vi "ReadSetLabelPosition__slk_mt.vi"(8 "error in (no error)":errorcluster, 11 "refnum in":T1) -> (0 "error out":errorcluster, 2 "set label position configure":T2={"Control Label Position"="Left Middle", "Indicator Label Position"="Right Middle", "Apply to All"=FALSE}, 3 "refnum out":T1)   [LabVIEW 2012, in "Lazyboots Menu Tool.lvlib"]
doc: "Gets configure datum of Set Label Position.\n\n<b>[Set Label Position]</b>\nControl Label Position = \"Left Middle\"\nIndicator Label Position = \"Right Middle\"\nApply to All = \"FALSE\""
uses:
  Library/Lazyboots Menu Tool.lvlib
  <vilib>/Utility/config.llb/NI_LVConfig.lvlib
  <vilib>/Utility/config.llb/Read Key (String).vi
  TypeDef/TypeDef_SetLabelPositionConfigure__slk_mt.ctl
  <vilib>/Utility/config.llb/Read Key (Boolean).vi
  <vilib>/Utility/config.llb/Config Data RefNum.ctl
panel:
  # "ReadSetLabelPosition__slk_mt.vi\nGets configure datum of Set Label Position.\n\nNOTICE -- YOU MUST LEAVE THIS NOTICE IN PLACE.\n\nCopyright (c) 2011, LIANG LIU Shawn.Liu.cn@gmail.com\nAll rights reserved.\n\nRedistribution and use in source and binary forms, with or without modification, are permitted provided that the following conditions are met:\n-Redistributions of source code must retain the above copyright notice, this list of conditions and the following disclaimer.\n-Redistributions in binary form must reproduce the above copyright notice, this list of conditions and the following disclaimer in the documentation and/or other materials provided with the distribution.\n-Neither the name of the eLp nor the names of its contributors may be used to endorse or promote products derived from this software without specific prior written permission.\n\nTHIS SOFTWARE IS PROVIDED BY THE COPYRIGHT HOLDERS AND CONTRIBUTORS \"AS IS\" AND ANY EXPRESS OR IMPLIED WARRANTIES, INCLUDING, BUT NOT LIMITED TO, THE IMPLIED WARRANTIES OF MERCHANTABILITY AND FITNESS FOR A PARTICULAR PURPOSE ARE DISCLAIMED. IN NO EVENT SHALL THE COPYRIGHT HOLDER OR CONTRIBUTORS BE LIABLE FOR ANY DIRECT, INDIRECT, INCIDENTAL, SPECIAL, EXEMPLARY, OR CONSEQUENTIAL DAMAGES (INCLUDING, BUT NOT LIMITED TO, PROCUREMENT OF SUBSTITUTE GOODS OR SERVICES; LOSS OF USE, DATA, OR PROFITS; OR BUSINESS INTERRUPTION) HOWEVER CAUSED AND ON ANY THEORY OF LIABILITY, WHETHER IN CONTRACT, STRICT LIABILITY, OR TORT (INCLUDING NEGLIGENCE OR OTHERWISE) ARISING IN ANY WAY OUT OF THE USE OF THIS SOFTWARE, EVEN IF ADVISED OF THE POSSIBILITY OF SUCH DAMAGE."
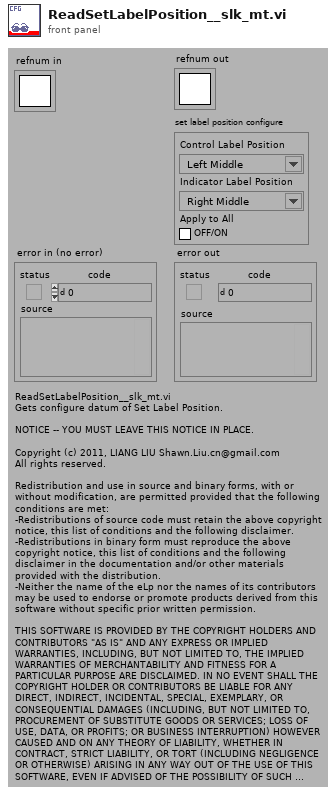
[diagram p1: front panel]
types:
  T1 = typedef "NI_LVConfig.lvlib/Config Data RefNum.ctl" = refnum<k1>
  T2 = typedef "Lazyboots Menu Tool.lvlib/TypeDef_SetLabelPositionConfigure__slk_mt.ctl" = cluster{"Control Label Position":string, "Indicator Label Position":string, "Apply to All":bool}
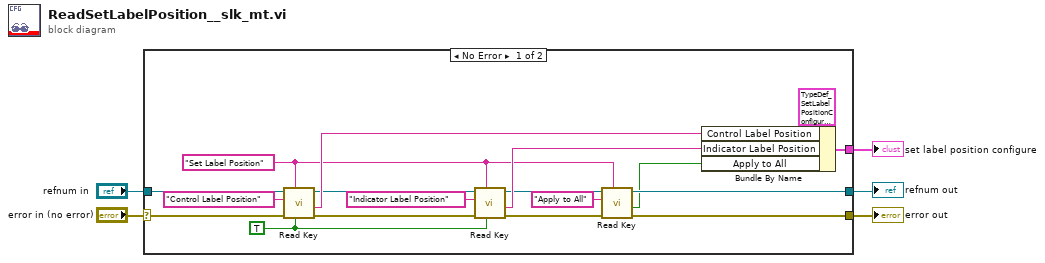
[diagram p0: block diagram]
diagram:
  n1 = case shown="No Error" "error in (no error)" {
    selector: "error in (no error)" -> [w15 w25]
    tunnel: [w16 _] -> w5
    tunnel: [w7 w25] -> w4
    tunnel: "refnum in" -> [w14 w24]
    tunnel: [w11 w24] -> w1
    frame No Error {
      w22 = TRUE ("read raw string? (F)")
      w10 = "Set Label Position" ("section")
      n2 = call-poly <vilib>:"Read Key.vi"("read raw string? (F)"=w22, "section"=w10, "error in (no error)"=w15, "key"="Control Label Position", "refnum"=w14) -> ("error out"=w23:errorcluster, "value"=w18:string, "refnum out"=w12:T1)  [unwired: 3 in, 1 out]
      n3 = call-poly <vilib>:"Read Key.vi"("read raw string? (F)"=w22, "section"=w10, "error in (no error)"=w23, "key"="Indicator Label Position", "refnum"=w12) -> ("error out"=w8:errorcluster, "value"=w17:string, "refnum out"=w13:T1)  [unwired: 3 in, 1 out]
      n4 = call-poly <vilib>:"Read Key.vi"("section"=w10, "error in (no error)"=w8, "key"="Apply to All", "refnum"=w13) -> ("error out"=w7:errorcluster, "value"=w6:bool, "refnum out"=w11:T1)  [unwired: 4 in, 1 out]
      n5 = Bundle By Name(cluster=T2 {"Control Label Position"="Left Middle", "Indicator Label Position"="Right Middle", "Apply to All"=FALSE} ("Set Label Position Configure"), "Control Label Position"=w18, "Indicator Label Position"=w17, "Apply to All"=w6) -> (w16:T2)
    }
    frame Error {
    }
  }
  "set label position configure" <- w5
  "error out" <- w4
  "refnum out" <- w1
